vi "Digital Pulse Generation (with PXIe-6624 Counter).vi"() -> ()   [LabVIEW 2019]
uses:
  <vilib>/Utility/error.llb/DialogType.ctl
  <vilib>/DAQmx/create/channels.llb/DAQmx Create Channel (CO-Pulse Generation-Time).vi
  <vilib>/DAQmx/configure/timing.llb/DAQmx Timing (Implicit).vi
  <resource>/objmgr/daqmx.rc
panel:
  out "CO.Pulse.Term":tag
  out "CO.CtrTimebaseSrc":tag
  out "CO.CtrTimebaseRate 2":dbl format="%#_6f"
  out "SampQuant.SampPerChan":dbl
  out "CO.Pulse.LowTime":dbl
  out "CO.Pulse.HighTime":dbl
  in  "low time":dbl=0.01 format="%#.8f"
  out "Frequency":dbl
  out "Period":dbl
  in  "PPR":dbl=18.0
  in  "RPM":dbl
  in  "Counter to Output with":tag="Dev1/ctr0"
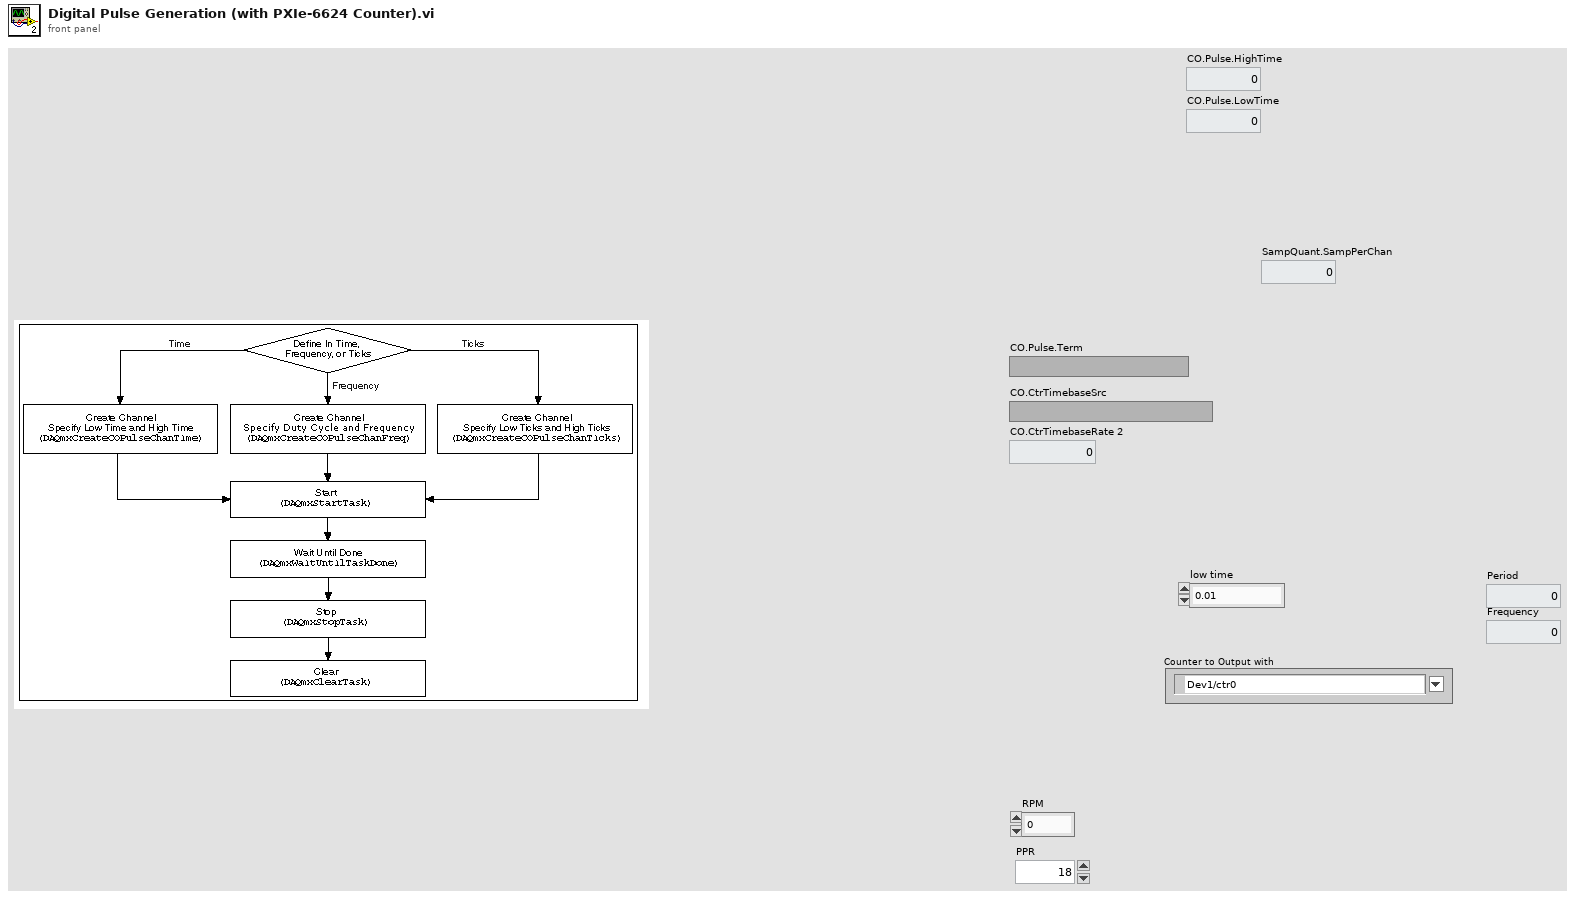
[diagram p1: front panel]
types:
  T1 = typedef "DialogType.ctl" = u16
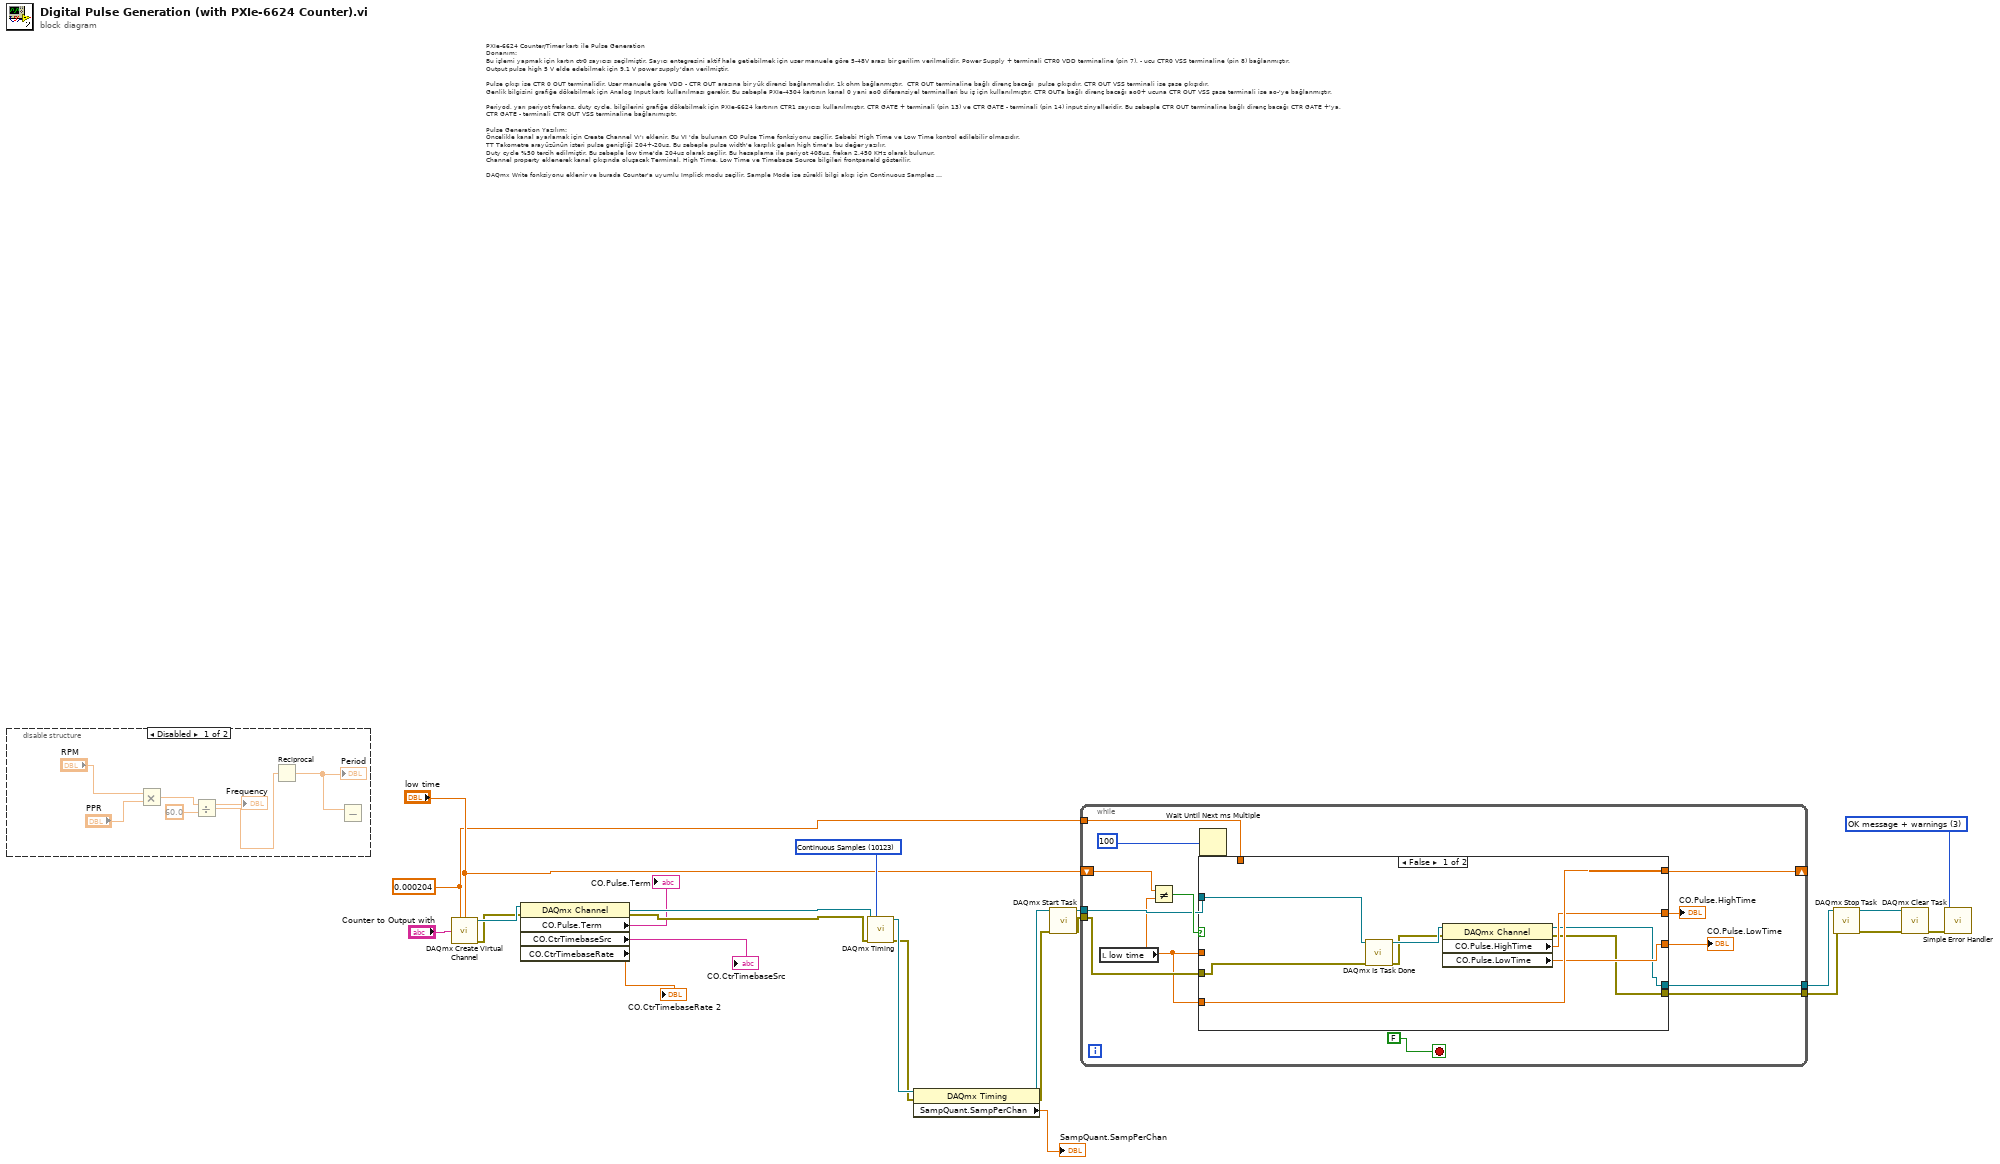
[diagram p0: block diagram]
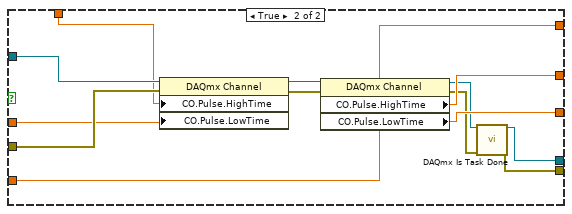
[diagram p3: hidden frame]
diagram:
  w8 = 0.000204 ("high time")
  w18 = T1 3 items=["no dialog", "OK message", "continue or stop message", "OK message + warnings", "continue/stop + warnings"] ("type of dialog (OK msg:1)")
  w21 = 10123 items=["Finite Samples"=10178, "Continuous Samples"=10123, "Hardware Timed Single Point"=12522] ("sample mode")
  # "PXIe-6624 Counter/Timer kartı ile Pulse Generation\nDonanım:\nBu işlemi yapmak için kartın ctr0 sayıcısı seçilmiştir. Sayıcı entegresini aktif hale getiebilmek için user manuele göre 5-48V arası bir gerilim verilmelidir. Power Supply + terminali CTR0 VDD terminaline (pin 7), - ucu CTR0 VSS terminaline (pin 8) bağlanmıştır. \nOutput pulse high 5 V elde edebilmek için 9.1 V power supply'dan verilmiştir. \n\nPulse çıkışı ise CTR 0 OUT terminalidir. User manuele göre VDD - CTR OUT arasına bir yük direnci bağlanmalıdır. 1k ohm bağlanmıştır.  CTR OUT terminaline bağlı direnç bacağı  pulse çıkışıdır. CTR OUT VSS terminali ise şase çıkışıdır.\nGenlik bilgisini grafiğe dökebilmek için Analog Input kartı kullanılması gerekir. Bu sebeple PXIe-4304 kartının kanal 0 yani ao0 diferansiyel terminalleri bu iş için kullanılmıştır. CTR OUTa bağlı direnç bacağı ao0+ ucuna CTR OUT VSS şase terminali ise ao-'ye bağlanmıştır.\n\nPeriyod, yarı periyot frekans, duty cycle, bilgilerini grafiğe dökebilmek için PXIe-6624 kartının CTR1 sayıcısı kullanılmıştır. CTR GATE + terminali (pin 13) ve CTR GATE - terminali (pin 14) input sinyalleridir. Bu sebeple CTR OUT terminaline bağlı direnç bacağı CTR GATE +'ya,\nCTR GATE - terminali CTR OUT VSS terminaline bağlanımışıtr. \n\nPulse Generation Yazılım:\nÖncelikle kanal ayarlamak için Create Channel Vı'ı eklenir. Bu VI 'da bulunan CO Pulse Time fonksiyonu seçilir. Sebebi High Time ve Low Time kontrol edilebilir olmasıdır. \nTT Takometre arayüzünün isteri pulse genişliği 204+-20us. Bu sebeple pulse width'e karşılık gelen high time'a bu değer yazılır. \nDuty cycle %50 tercih edilmiştir. Bu sebeple low time'da 204us olarak seçilir. Bu hesaplama ile periyot 408us, frekan 2.450 KHz olarak bulunur.\nChannel property eklenerek kanal çıkışında oluşacak Terminal, High Time, Low Time ve Timebase Source bilgileri frontpaneld gösterilir.\n\nDAQmx Write fonksiyonu eklenir ve burada Counter'a uyumlu Implick modu seçilir. Sample Mode ise sürekli bilgi akışı için Continuous Samples seçilir.\nGörevi başlatmak için Start VI'ı eklenir.\nStop btonuna basana kadar dönecek DAQmx is Task Done Vı'ı ile pulse üretimi gerçekleştirilir."
  n1 = disable-structure shown="Disabled" {
    frame Disabled {
      n2 = Multiply(x="RPM", y="PPR") -> (x*y=w30:dbl)
      n3 = Divide(x=w30, y=60.0) -> (x/y=w27:dbl)
      "Frequency" <- w27
      n4 = Reciprocal(x=w27) -> (1/x=w25:dbl)
      "Period" <- w25
      n5 = Subtract(x=w25) -> ()  [unwired: 1 in, 1 out]
    }
    frame Enabled {
    }
  }
  n6 = call-poly <vilib>:"DAQmx Create Virtual Channel.vi"("high time"=w8, "low time"="low time", "counter"="Counter to Output with") -> ("task out"=w5:refnum<k21>, "error out"=w4:errorcluster)  [unwired: 11 in]
  n7 = property class="DAQmx Channel"(reference=w5, error in=w4) -> (reference out=w22:refnum<k21>, error out=w23:errorcluster, "CO.Pulse.Term"=→"CO.Pulse.Term":tag, "CO.CtrTimebaseSrc"=→"CO.CtrTimebaseSrc":tag, "CO.CtrTimebaseRate"=→"CO.CtrTimebaseRate 2":dbl)
  n8 = call-poly <vilib>:"DAQmx Timing.vi"("task/channels in"=w22, "sample mode"=w21, "error in"=w23) -> ("task out"=w17:refnum<k21>, "error out"=w16:errorcluster)  [unwired: 11 in]
  n9 = property class="DAQmx Timing"(reference=w17, error in=w16) -> (reference out=w15:refnum<k21>, error out=w14:errorcluster, "SampQuant.SampPerChan"=→"SampQuant.SampPerChan":dbl)
  n10 = call <vilib>:"DAQmx Start Task.vi"("task/channels in"=w15, "error in"=w14) -> ("task out"=w20:refnum<k21>, "error out"=w12:errorcluster)  [unwired: 12 in]
  n11 = while {
    tunnel: w12 -> [w39]
    tunnel: w20 -> [w40]
    shift-right: [w35] -> _
    shift-left: "low time" -> [w37]
    tunnel: w8 -> [w38]
    tunnel: [w34] -> w7
    tunnel: [w33] -> w6
    stop <- FALSE stop-if-true
    n12 = local read "low time"() -> (w36:dbl)
    n13 = Not Equal?(x=w37, y=w36) -> (x != y?=w41:bool)
    n14 = case shown="False" w41 {
      tunnel: w40 -> [w52 w64]
      tunnel: w39 -> [w51 w63]
      tunnel: w38 -> [_ w59]
      tunnel: w36 -> [_ w60]
      tunnel: [w45 w62] -> w34
      tunnel: [w44 w61] -> w33
      tunnel: w36 -> [w50 w65]
      tunnel: [w50 w65] -> w35
      tunnel: [w47 w56] -> w32
      tunnel: [w46 w55] -> w31
      frame False {
        n15 = call <vilib>:"DAQmx Is Task Done.vi"("task/channels in"=w52, "error in"=w51) -> ("task out"=w49:refnum<k21>, "error out"=w48:errorcluster)  [unwired: 11 in, 1 out]
        n16 = property class="DAQmx Channel"(reference=w49, error in=w48) -> (reference out=w45:refnum<k21>, error out=w44:errorcluster, "CO.Pulse.HighTime"=w47:dbl, "CO.Pulse.LowTime"=w46:dbl)
      }
      frame True {
        n17 = property class="DAQmx Channel"(reference=w64, error in=w63, "CO.Pulse.HighTime"=w59, "CO.Pulse.LowTime"=w60) -> (reference out=w58:refnum<k21>, error out=w57:errorcluster)
        n18 = property class="DAQmx Channel"(reference=w58, error in=w57) -> (reference out=w54:refnum<k21>, error out=w53:errorcluster, "CO.Pulse.HighTime"=w56:dbl, "CO.Pulse.LowTime"=w55:dbl)
        n19 = call <vilib>:"DAQmx Is Task Done.vi"("task/channels in"=w54, "error in"=w53) -> ("task out"=w62:refnum<k21>, "error out"=w61:errorcluster)  [unwired: 11 in, 1 out]
      }
    }
    "CO.Pulse.HighTime" <- w32
    "CO.Pulse.LowTime" <- w31
    n20 = Wait Until Next ms Multiple(millisecond multiple=100) -> ()  [unwired: 1 out]
  }
  n21 = call <vilib>:"DAQmx Stop Task.vi"("task/channels in"=w7, "error in"=w6) -> ("task out"=w11:refnum<k21>, "error out"=w10:errorcluster)  [unwired: 12 in]
  n22 = call <vilib>:"DAQmx Clear Task.vi"("task in"=w11, "error in"=w10) -> ("error out"=w19:errorcluster)  [unwired: 13 in]
  n23 = call <vilib>:"Simple Error Handler.vi"("type of dialog (OK msg:1)"=w18, "error in (no error)"=w19) -> ()  [unwired: 3 in, 5 out]
